vi "Initialize Sink.vi"(11 "LVQueue Sink in":refnum<class "LVQueue Sink.lvclass">) -> (0 "error out":errorcluster, 3 "LVQueue Sink out":refnum<class "LVQueue Sink.lvclass">)   [LabVIEW 2017, in "LVQueue Sink.lvclass"]
uses:
  LVQueue Sink.lvclass
  LVQueue Sink.lvclass/LVQueue Sink.ctl
  <vilib>/Utility/error.llb/Error Cluster From Error Code.vi
  <vilib>/ErrorRing/Error Ring.xnode
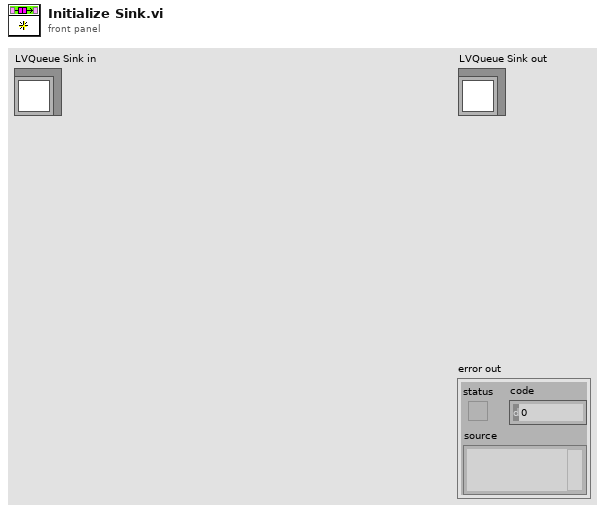
[diagram p1: front panel]
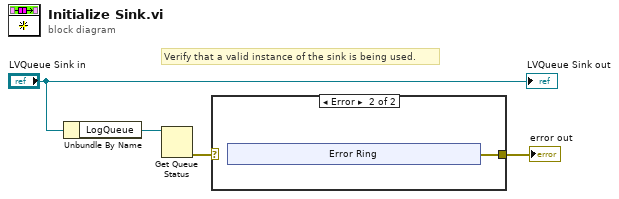
[diagram p0: block diagram]
diagram:
  # "Verify that a valid instance of the sink is being used."
  n1 = Unbundle By Name("LVQueue Sink in") -> ("LogQueue"=w3:refnum<queue>)
  n2 = Get Queue Status(queue=w3) -> (error out=w2:errorcluster)  [unwired: 2 in, 7 out]
  n3 = case shown="Error" w2 {
    selector: w2 -> [w5 _]
    tunnel: [w5 w6] -> w1
    frame No Error {
    }
    frame Error {
      n4 = xnode "Error Ring"() -> ("error out"=w6:errorcluster)
    }
  }
  "error out" <- w1
  "LVQueue Sink out" <- "LVQueue Sink in"
